vi "生产调试用上位机.vi"() -> ()   [LabVIEW 2016]
uses:
  <vilib>/Utility/miscctls.llb/LVPointTypeDef.ctl
  <vilib>/Utility/config.llb/NI_LVConfig.lvlib
panel:
  in  "报警查询":bool
  in  "日志查询":bool
  in  "主页按钮":bool
  in  "数据查询":bool
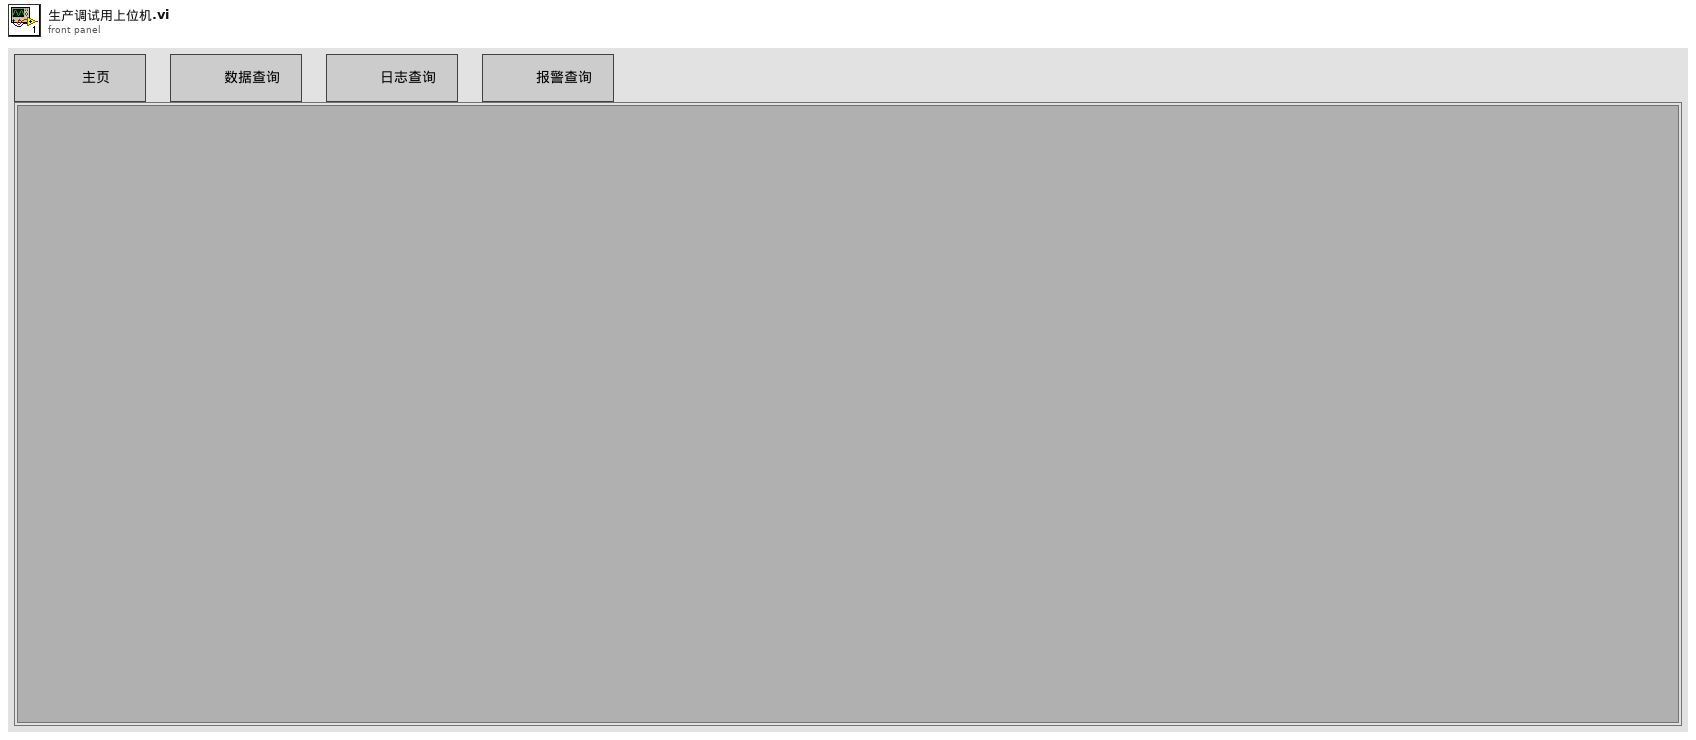
[diagram p1: front panel]
types:
  T1 = typedef "LVPointTypeDef.ctl" = cluster{"Horizontal":i16, "Vertical":i16}
  T2 = typedef "NI_LVConfig.lvlib/Config Data RefNum.ctl" = refnum<k1>
  T3 = enum32{"Bad", "Idle", "Run top level", "Running"}
  T4 = typedef "imagedata.ctl" = cluster{"image type":i32, "image depth":i32, "image":u8[], "mask":u8[], "colors":u32[], "Rectangle":cluster{"left":i16, "top":i16, "right":i16, "bottom":i16}}
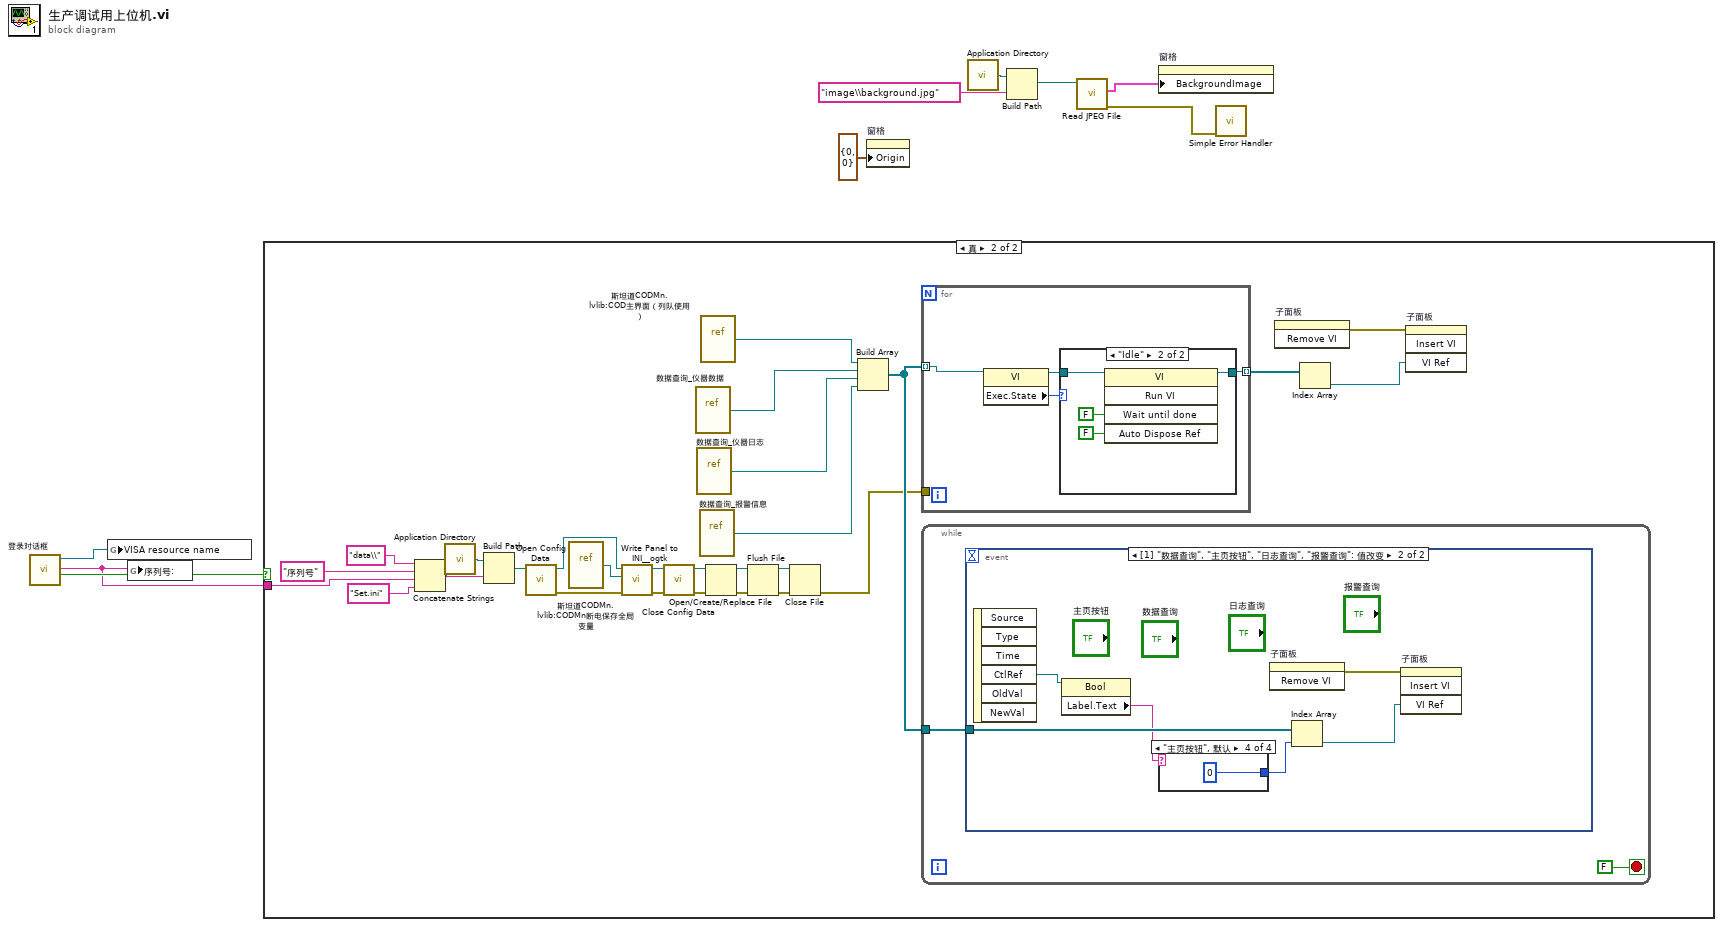
[diagram p0: block diagram]
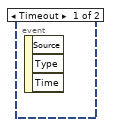
[diagram p4: hidden frame]
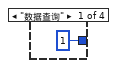
[diagram p5: hidden frame]
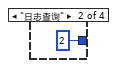
[diagram p6: hidden frame]
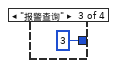
[diagram p7: hidden frame]
diagram:
  n1 = call "登录对话框.vi"() -> ("输出"=w4:bool, "序列号"=w1:string, "串口号"=w3:refnum<visa-resource-name>)  [unwired: 7 in]
  n2 = global write "CODMn断电保存全局变量.vi" "VISA resource name"(w3) -> ()
  n3 = global write "COD内部交互全局.vi" "序列号:"(w1) -> ()
  n4 = case shown="真" w4 {
    tunnel: w1 -> [_ w27]
    frame False {
    }
    frame True {
      n5 = Concatenate Strings("data\\" ("字符串"), "序列号" ("字符串"), w27, "Set.ini" ("名称或相对路径")) -> (w13:string)
      n6 = call <vilib>:"Application Directory.vi"() -> ("Application Directory"=w14:path)
      n7 = Build Path(base path=w14, name or relative path=w13) -> (appended path=w15:path)
      n8 = call <vilib>:"Open Config Data.vi"("configuration file path"=w15) -> ("error out"=w19:errorcluster, "refnum"=w16:T2)  [unwired: 8 in, 1 out]
      n9 = vi-ref "斯坦道CODMn.lvlib:CODMn断电保存全局变量.vi"() -> (w17:refnum<vi>)
      n10 = call <userlib>:"Write Panel to INI__ogtk.vi"("error in (no error)"=w19, "VI ref"=w17, "refnum"=w16) -> ("error out"=w20:errorcluster, "refnum out"=w18:T2)  [unwired: 7 in]
      n11 = call <vilib>:"Close Config Data.vi"("error in (no error)"=w20, "refnum"=w18) -> ("error out"=w25:errorcluster, "file path"=w26:path)  [unwired: 8 in]
      n12 = vi-ref "数据查询_仪器数据.vi"() -> (w35:refnum<vi>)
      n13 = vi-ref "数据查询_仪器日志.vi"() -> (w10:refnum<vi>)
      n14 = vi-ref "数据查询_报警信息.vi"() -> (w11:refnum<vi>)
      n15 = vi-ref "斯坦道CODMn.lvlib:COD主界面（列队使用）.vi"() -> (w36:refnum<vi>)
      n16 = Open/Create/Replace File(file path (use dialog)=w26, error in=w25) -> (refnum out=w22:refnum<file>, error out=w21:errorcluster)  [unwired: 4 in, 1 out]
      n17 = Flush File(refnum=w22, error in=w21) -> (refnum out=w23:refnum<file>, error out=w24:errorcluster)
      n18 = Close File(refnum=w23, error in=w24) -> (error out=w12:errorcluster)  [unwired: 1 out]
      n19 = Build Array(w36, w35, w10, w11) -> (w31:refnum<vi>[])
      n20 = for {
        tunnel: [w38] -> w33 mode=indexing
        tunnel: w31 -> [w37] mode=indexing
        tunnel: w12 -> [_]
        n21 = property class="VI"(reference=w37) -> (reference out=w39:refnum<vi>, "Exec.State"=w40:T3)  [unwired: 1 in, 1 out]
        n22 = case shown="\"Idle\"" w40 {
          tunnel: w39 -> [w41 w43]
          tunnel: [w41 w42] -> w38
          frame "Bad", Default {
          }
          frame "Idle" {
            n23 = invoke class="VI" method="Run VI"(reference=w43, "Wait until done"=FALSE ("结束前等待"), "Auto Dispose Ref"=FALSE ("自动销毁引用")) -> (reference out=w42:refnum<vi>)  [unwired: 2 in, 4 out]
          }
        }
      }
      n24 = while {
        tunnel: w31 -> [w46]
        stop <- FALSE stop-if-true
        n25 = event shown="[1] \"数据查询\", \"主页按钮\", \"日志查询\", \"报警查询\": 值改变" {
          selector: _ -> [_ _]
          dyn-events: _ -> [_ _]
          timeout: _ -> [_ _]
          tunnel: w46 -> [_ w51]
          event Timeout {
            n26 = event-data() -> ()  [unwired: 1 in, 3 out]
          }
          event "数据查询", "主页按钮", "日志查询", "报警查询": Value Change {
            n27 = event-data() -> ("CtlRef"=w50:refnum<vi>)  [unwired: 1 in, 5 out]
            n28 = property class="Bool"(reference=w50) -> ("Label.Text"=w49:string)  [unwired: 1 in, 2 out]
            n29 = case shown="\"主页按钮\", 默认" w49 {
              tunnel: [1 ("索引") 2 ("索引") 3 ("索引") 0 ("索引")] -> w48
              frame "数据查询" {
              }
              frame "日志查询" {
              }
              frame "报警查询" {
              }
              frame "主页按钮", Default {
              }
            }
            n30 = invoke on="子面板" class="SubPnl" method="Remove VI"() -> (error out=w52:errorcluster)  [unwired: 3 in, 2 out]
            n31 = Index Array(array=w51, index=w48) -> (element=w53:refnum<vi>)
            n32 = invoke on="子面板" class="SubPnl" method="Insert VI"(error in=w52, "VI Ref"=w53) -> ()  [unwired: 2 in, 4 out]
          }
        }
      }
      n33 = invoke on="子面板" class="SubPnl" method="Remove VI"() -> (error out=w34:errorcluster)  [unwired: 3 in, 2 out]
      n34 = Index Array(array=w33) -> (element=w32:refnum<vi>)  [unwired: 1 in]
      n35 = invoke on="子面板" class="SubPnl" method="Insert VI"(error in=w34, "VI Ref"=w32) -> ()  [unwired: 2 in, 4 out]
    }
  }
  n36 = property on="窗格" class="Pane"("Origin"=T1 {"Horizontal"=0, "Vertical"=0} ("原点")) -> ()  [unwired: 2 in, 2 out]
  n37 = call <vilib>:"Application Directory.vi"() -> ("Application Directory"=w9:path)
  n38 = Build Path(base path=w9, name or relative path="image\\background.jpg" ("名称或相对路径")) -> (appended path=w7:path)
  n39 = call <vilib>:"Read JPEG File.vi"("path to JPEG file"=w7) -> ("error out"=w5:errorcluster, "image data"=w6:T4)  [unwired: 8 in, 1 out]
  n40 = property on="窗格" class="Pane"("BackgroundImage"=w6) -> ()  [unwired: 2 in, 2 out]
  n41 = call <vilib>:"Simple Error Handler.vi"("error in (no error)"=w5) -> ()  [unwired: 4 in, 5 out]
